vi "FRCts20_EspEngine_DebugInitSearchBrowser.vi"(8 "error in (no error)":errorcluster, 9 "select-choice-location":string, 10 "select-choice-software":T1, 11 "httpRequestID":u32) -> (0 "error out":errorcluster, 2 "SearchBrowser":T3, 3 "httpRequestID out":u32)   [LabVIEW 2014, in "FRCts20_EspEngine.lvlib"]
uses:
  FRCts20_EspEngine.lvlib
  <vilib>/wsapi/NI_WebServices.lvlib
  TypeDefs/FRCts20_EspEngine_SearchBrowser.ctl
  <vilib>/wsapi/subVIs/Write Single Session Variable.vi
  Backend/source/VI Source/FRCts20_Backend_API/FRCts20_Backend_API_Command_EventRoot.ctl
  Backend/source/VI Source/FRCts20_Backend_API/FRCts20_Backend_API_SW.ctl
  Backend/source/VI Source/FRCts20_Backend_API/FRCts20_Backend_API_EventRoot.ctl
panel:
  in  "EventRoot In":T2={"Event"=[{"Event Index"=0, "EventID"=0, "EventSubtype"="", "EventSubtypeID"=0, "DistrictCode"="", "DistrictID"=0, "Event Name"="NYC", "Venue"="", "City"="", "StateProvince"="", "Country"="", "Start Time"=timestamp(0 s since 1904-01-01), "End Time"=timestamp(0 s since 1904-01-01), "Year"=0, "NumberOfTeams"=0, "URLTeamlist"="", "EventCode"="", "OpenIssues"=0, "IsLive"=TRUE}, {"Event Index"=0, "EventID"=0, "EventSubtype"="", "EventSubtypeID"=0, "DistrictCode"="", "DistrictID"=0, "Event Name"="SF", "Venue"="", "City"="", "StateProvince"="", "Country"="", "Start Time"=timestamp(0 s since 1904-01-01), "End Time"=timestamp(0 s since 1904-01-01), "Year"=0, "NumberOfTeams"=0, "URLTeamlist"="", "EventCode"="", "OpenIssues"=0, "IsLive"=TRUE}, {"Event Index"=0, "EventID"=0, "EventSubtype"="", "EventSubtypeID"=0, "DistrictCode"="", "DistrictID"=0, "Event Name"="OKC", "Venue"="", "City"="", "StateProvince"="", "Country"="", "Start Time"=timestamp(0 s since 1904-01-01), "End Time"=timestamp(0 s since 1904-01-01), "Year"=0, "NumberOfTeams"=0, "URLTeamlist"="", "EventCode"="", "OpenIssues"=0, "IsLive"=TRUE}], "APIReturn"=""}
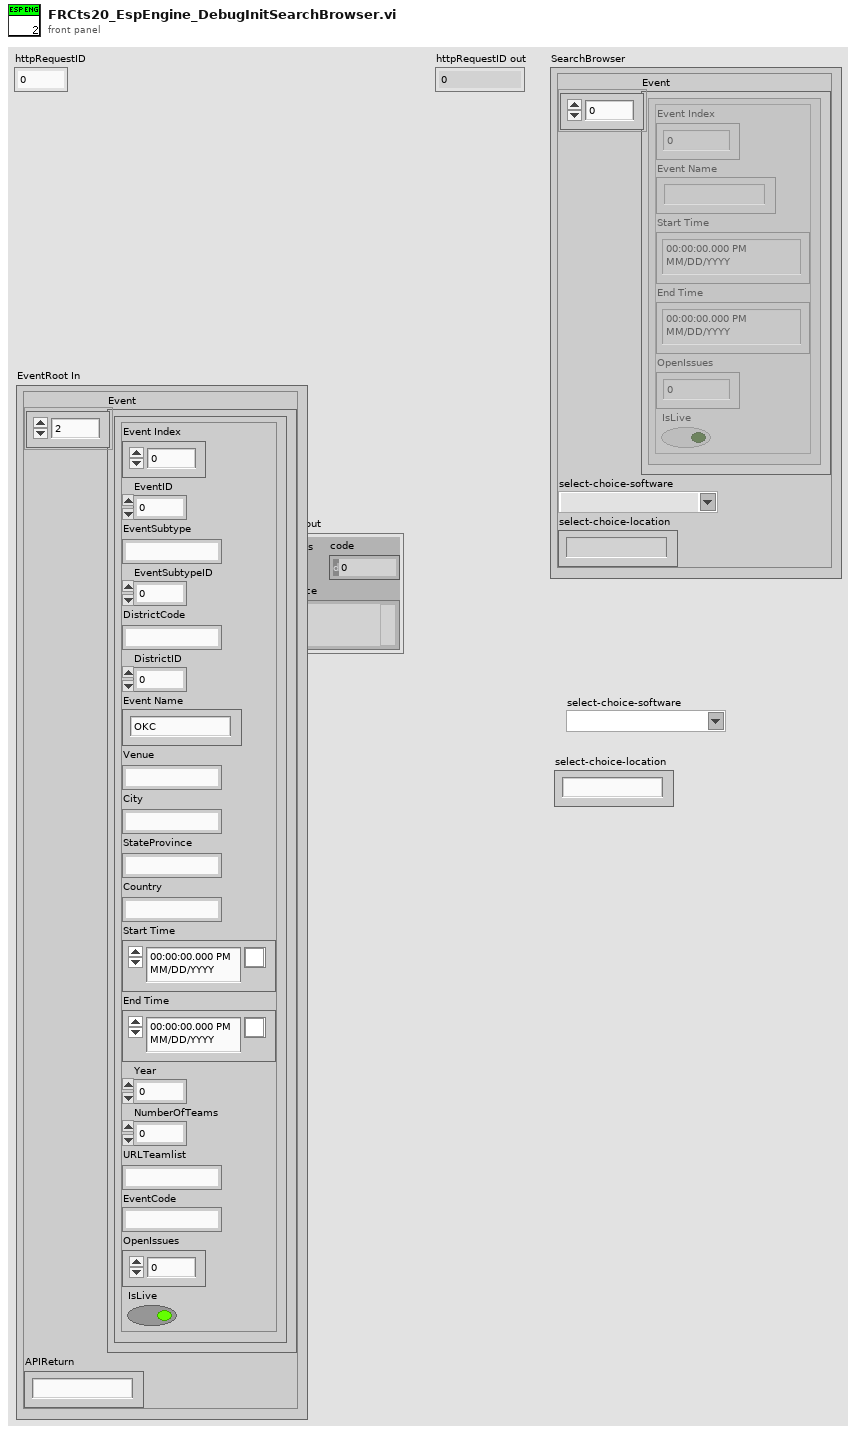
[diagram p1: front panel]
types:
  T1 = typedef "FRCts20_Backend_API.lvlib/FRCts20_Backend_API_SW.ctl" = string
  T2 = typedef "FRCts20_Backend_API.lvlib/FRCts20_Backend_API_EventRoot.ctl" = cluster{"Event":cluster{"Event Index":u32, "EventID":u32, "EventSubtype":string, "EventSubtypeID":u32, "DistrictCode":string, "DistrictID":u32, "Event Name":string, "Venue":string, "City":string, "StateProvince":string, "Country":string, "Start Time":timestamp, "End Time":timestamp, "Year":u32, "NumberOfTeams":u32, "URLTeamlist":string, "EventCode":string, "OpenIssues":u8, "IsLive":bool}[], "APIReturn":string}
  T3 = typedef "FRCts20_EspEngine.lvlib/FRCts20_EspEngine_SearchBrowser.ctl" = cluster{"Event":cluster{"Event Index":u32, "Event Name":string, "Start Time":timestamp, "End Time":timestamp, "OpenIssues":u8, "IsLive":bool}[], "select-choice-software":string, "select-choice-location":string}
  T4 = typedef "FRCts20_Backend_API.lvlib/FRCts20_Backend_API_Command_EventRoot.ctl" = string
  T5 = cluster{"Event Index":u32, "EventID":u32, "EventSubtype":string, "EventSubtypeID":u32, "DistrictCode":string, "DistrictID":u32, "Event Name":string, "Venue":string, "City":string, "StateProvince":string, "Country":string, "Start Time":timestamp, "End Time":timestamp, "Year":u32, "NumberOfTeams":u32, "URLTeamlist":string, "EventCode":string, "OpenIssues":u8, "IsLive":bool}[]
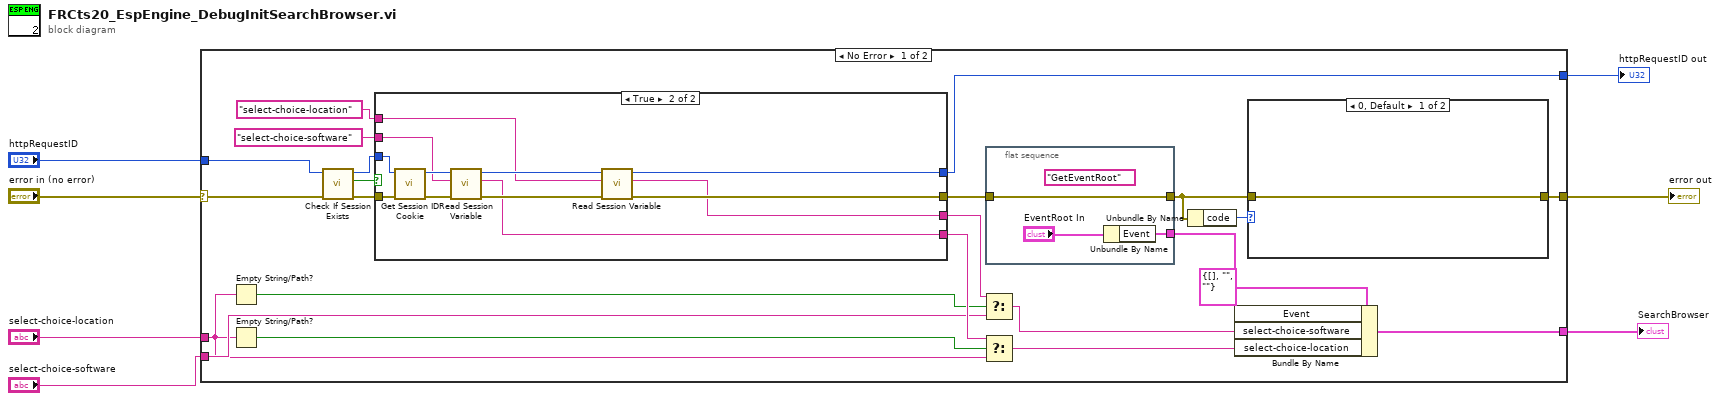
[diagram p0: block diagram]
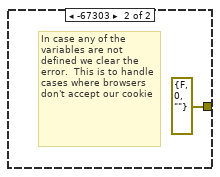
[diagram p2: hidden frame]
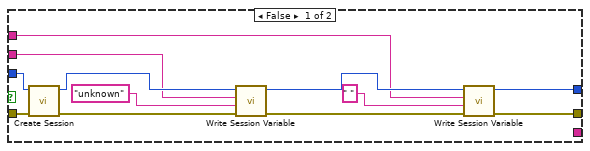
[diagram p3: hidden frame]
diagram:
  n1 = case shown="No Error" "error in (no error)" {
    selector: "error in (no error)" -> [w25 w60]
    tunnel: [w17 w60] -> w7
    tunnel: [w26 _] -> w5
    tunnel: "httpRequestID" -> [w24 _]
    tunnel: [w22 _] -> w3
    tunnel: "select-choice-software" -> [w11 _]
    tunnel: "select-choice-location" -> [w9 _]
    frame No Error {
      n2 = Empty String/Path?(string/path=w9) -> (empty?=w13:bool)
      n3 = Empty String/Path?(string/path=w9) -> (empty?=w14:bool)
      n4 = call <vilib>:"Check If Session Exists.vi"("error in (no error)"=w25, "httpRequestID"=w24) -> ("error out"=w30:errorcluster, "session exists?"=w29:bool, "httpRequestID out"=w28:u32)  [unwired: 7 in]
      n5 = case shown="True" w29 {
        tunnel: w28 -> [w44 w56]
        tunnel: w30 -> [w43 w55]
        tunnel: [w36 w51] -> w23
        tunnel: [w40 w49] -> w22
        tunnel: "select-choice-software" ("key") -> [w35 w48]
        tunnel: "select-choice-location" ("key") -> [w34 w47]
        tunnel: [_ w46] -> w15
        tunnel: [_ w45] -> w12
        frame False {
          n6 = call <vilib>:"Create Session.vi"("error in (no error)"=w43, "httpRequestID"=w44) -> ("error out"=w38:errorcluster, "httpRequestID out"=w42:u32)  [unwired: 7 in, 1 out]
          n7 = call-poly <vilib>:"Write Session Variable.vi"("error in (no error)"=w38, "value"="unknown", "key"=w35, "httpRequestID"=w42) -> ("error out"=w37:errorcluster, "httpRequestID out"=w41:u32)  [unwired: 4 in, 2 out]
          n8 = call-poly <vilib>:"Write Session Variable.vi"("error in (no error)"=w37, "value"=" ", "key"=w34, "httpRequestID"=w41) -> ("error out"=w36:errorcluster, "httpRequestID out"=w40:u32)  [unwired: 4 in, 2 out]
        }
        frame True {
          n9 = call <vilib>:"Get Session ID Cookie.vi"("error in (no error)"=w55, "httpRequestID"=w56) -> ("error out"=w52:errorcluster, "httpRequestID out"=w50:u32)  [unwired: 7 in, 1 out]
          n10 = call <vilib>:"Read Session Variable.vi"("error in (no error)"=w52, "key"=w48, "httpRequestID"=w50) -> ("error out"=w53:errorcluster, "value"=w46:string, "httpRequestID out"=w54:u32)  [unwired: 6 in]
          n11 = call <vilib>:"Read Session Variable.vi"("error in (no error)"=w53, "key"=w47, "httpRequestID"=w54) -> ("error out"=w51:errorcluster, "value"=w45:string, "httpRequestID out"=w49:u32)  [unwired: 6 in]
        }
      }
      n12 = Select(t=w12, s=w13, f=w11) -> (s? t:f=w10:T1)
      n13 = Select(t=w15, s=w14, f=w9) -> (s? t:f=w8:string)
      n14 = flat-sequence {
        tunnel: w23 -> [w59]
        tunnel: [w59] -> w18
        tunnel: [w58] -> w16
        frame #0 {
          (unwired) T4 "GetEventRoot" ("Message")
          n15 = Unbundle By Name("EventRoot In") -> ("Event"=w58:T5)
        }
      }
      n16 = Unbundle By Name(w18) -> ("code"=w19:i32)
      n17 = Bundle By Name(cluster=T3 {"Event"=[], "select-choice-software"="", "select-choice-location"=""} ("SearchBrowser"), "Event"=w16, "select-choice-software"=w10, "select-choice-location"=w8) -> (w26:T3)
      n18 = case shown="0, Default" w19 {
        tunnel: [w31 errorcluster {"status"=FALSE, "code"=0, "source"=""} ("error out")] -> w17
        tunnel: w18 -> [w31 _]
        frame 0, Default {
        }
        frame -67303 {
          # "In case any of the variables are not defined we clear the error.  This is to handle cases where browsers don't accept our cookie"
        }
      }
    }
    frame Error {
    }
  }
  "error out" <- w7
  "SearchBrowser" <- w5
  "httpRequestID out" <- w3
